vi "runExperimentV2.vi"(8 "error in (no error)":errorcluster, 9 "runExperiment.Enum":enum16{"runListOnce", "loopOverList"}(ring), 10 "index":i32, 11 "ExperimentRunner in":refnum<class "ExperimentRunner.lvclass">) -> (0 "error out":errorcluster, 3 "ExperimentRunner out":refnum<class "ExperimentRunner.lvclass">)   [LabVIEW 2011, in "Views.lvlib" / "ExperimentControl.lvlib" / "ExperimentRunner.lvclass"]
uses:
  ExperimentRunner.lvclass
  ExperimentRunner.lvclass/ExperimentRunner.ctl
  Events/ExperimentControlEvents.lvclass
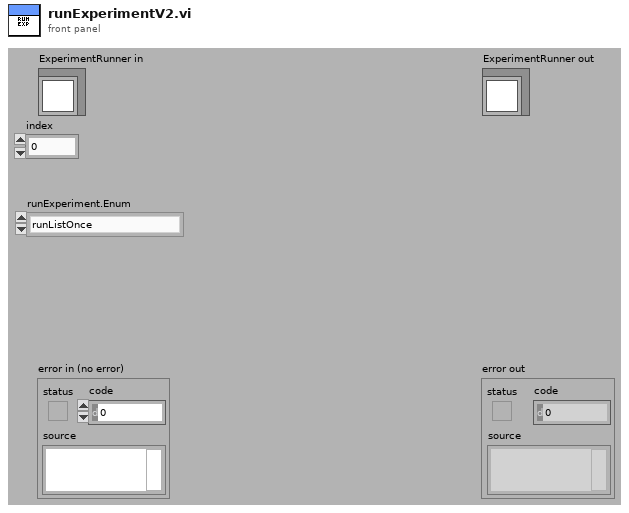
[diagram p1: front panel]
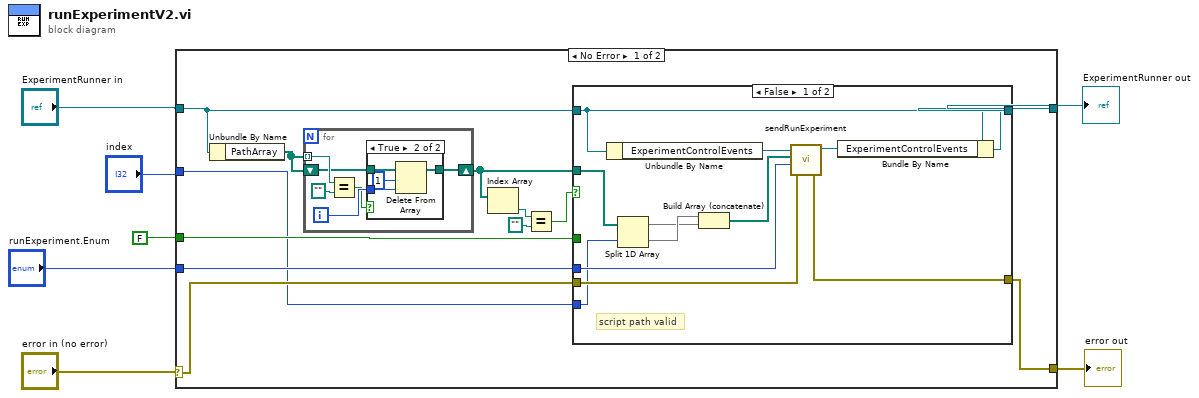
[diagram p0: block diagram]
diagram:
  n1 = case shown="No Error" "error in (no error)" {
    selector: "error in (no error)" -> [w16 w45]
    tunnel: [w18 w46] -> w5
    tunnel: "ExperimentRunner in" -> [w19 w46]
    tunnel: FALSE -> [w17 _]
    tunnel: "index" -> [w8 _]
    tunnel: [w15 w45] -> w4
    tunnel: "runExperiment.Enum" -> [w9 _]
    frame No Error {
      n2 = Unbundle By Name(w19) -> ("PathArray"=w14:path[])
      n3 = for {
        tunnel: w14 -> [w24] mode=indexing
        shift-right: [w22] -> w10
        shift-left: w14 -> [w23]
        i -> [w21]
        n4 = Equal?(x=w24, y=path "") -> (x = y?=w20:bool)
        n5 = case shown="True" w20 {
          tunnel: w23 -> [w26 w30]
          tunnel: [w26 w29] -> w22
          tunnel: w21 -> [_ w28]
          frame False {
          }
          frame True {
            n6 = Delete From Array(array=w30, length=1, index=w28) -> (array with subset deleted=w29:path[])  [unwired: 1 out]
          }
        }
      }
      n7 = Index Array(array=w10) -> (element=w12:path)  [unwired: 1 in]
      n8 = Equal?(x=w12, y=path "") -> (x = y?=w11:bool)
      n9 = case shown="False" w11 {
        tunnel: w19 -> [w42 w44]
        tunnel: [w41 w44] -> w18
        tunnel: w17 -> [_ _]
        tunnel: w16 -> [w37 w43]
        tunnel: [w38 w43] -> w15
        tunnel: w10 -> [w34 _]
        tunnel: w9 -> [w36 _]
        tunnel: w8 -> [w35 _]
        frame False {
          # "script path valid"
          n10 = Unbundle By Name(w42) -> ("ExperimentControlEvents"=w40:refnum<class "ExperimentControlEvents.lvclass">)
          n11 = Split 1D Array(array=w34, index=w35) -> (first subarray=w32:path[], second subarray=w33:path[])
          n12 = Build Array (concatenate)(w33, w32) -> (w31:path[])
          n13 = call "sendRunExperiment.vi"("error in (no error)"=w37, "runExperiment.Enum"=w36, "runExperiment.Array"=w31, "ExperimentControlEvents in"=w40) -> ("error out"=w38:errorcluster, "ExperimentControlEvents out"=w39:refnum<class "ExperimentControlEvents.lvclass">)  [unwired: 6 in]
          n14 = Bundle By Name(cluster=w42, "ExperimentControlEvents"=w39) -> (w41:refnum<class "ExperimentRunner.lvclass">)
        }
        frame True {
          # "empty script path"
        }
      }
    }
    frame Error {
    }
  }
  "error out" <- w4
  "ExperimentRunner out" <- w5
